vi "Parse Coords.vi"(8 "error in (no error)":errorcluster, 10 "Read Coordinates":path, 11 "Stage Actor.lvlib:Stage.lvclass":refnum<class "Stage.lvclass">) -> (0 "error out":errorcluster, 3 "Stage Actor.lvlib:Stage.lvclass":refnum<class "Stage.lvclass">)   [LabVIEW 2018, in "Stage Actor.lvlib" / "Stage.lvclass"]
uses:
  Stage.lvclass
  Stage.lvclass/Stage.ctl
  <vilib>/Utility/file.llb/Read Delimited Spreadsheet (string).vi
  Stage Actor.lvlib
  <instrlib>/Zaber A Series/Zaber A Series.lvlib
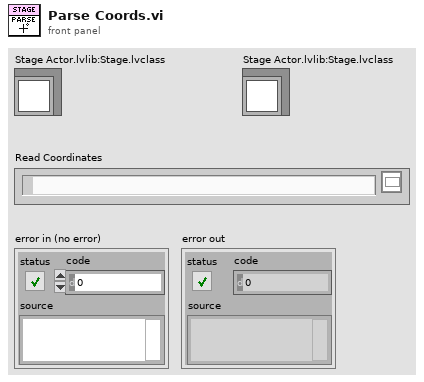
[diagram p1: front panel]
types:
  T1 = enum32{"invalid app kind", "Development System", "Run Time System", "Student Edition", "Embedded LabVIEW", "Evaluation", "Custom"}
  T2 = cluster{"XY":dbl[][], "Theta Phi":dbl[][], "Current Tool":i16[], "Speed":dbl[], "Feeder State":bool[], "Z":dbl[]}
  T3 = cluster{"Current Tool":i16, "Speed":dbl, "Feeder State":bool, "Z":dbl, "XY":dbl[], "Theta Phi":dbl[]}
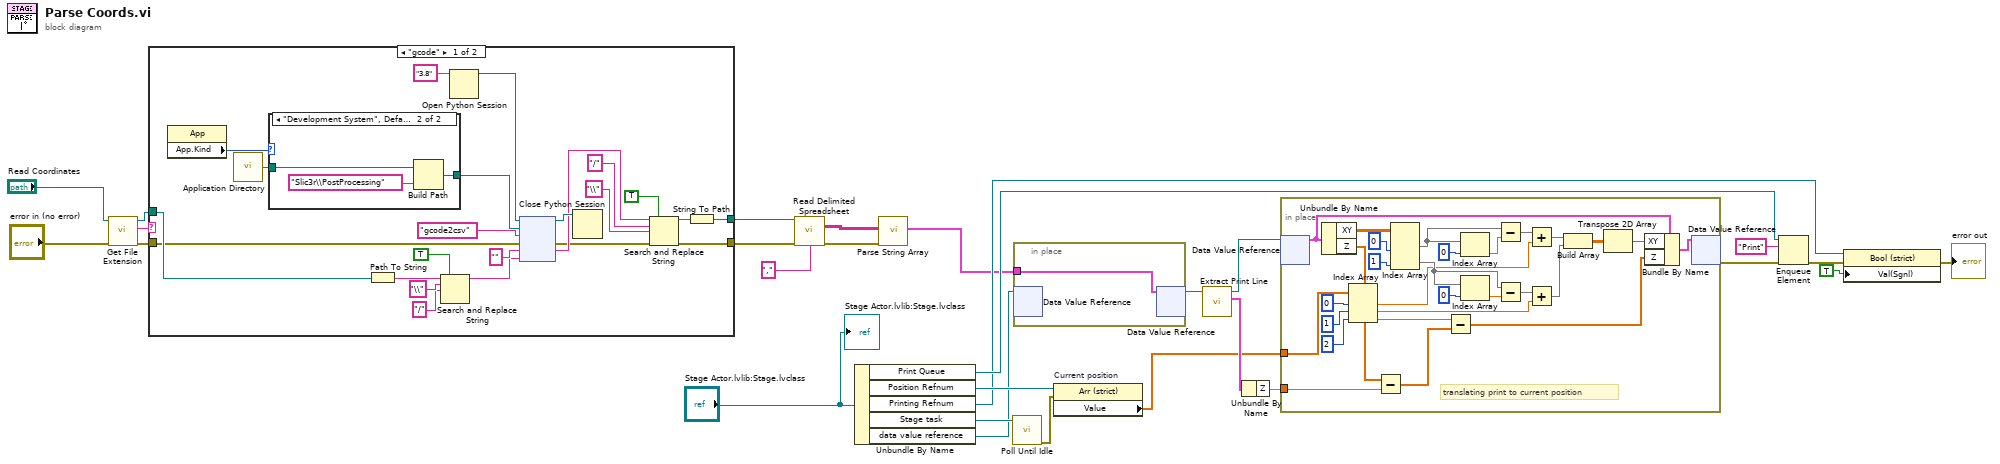
[diagram p0: block diagram]
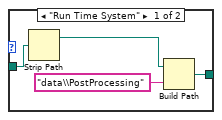
[diagram p2: hidden frame]
diagram:
  n1 = call <vilib>:"Get File Extension.vi"("error in (no error)"="error in (no error)", "file"="Read Coordinates") -> ("error out"=w19:errorcluster, "lowercase file extension"=w21:string, "dup file"=w20:path)  [unwired: 5 in, 2 out]
  n2 = case shown="\"gcode\"" w21 {
    tunnel: w20 -> [w48 w60]
    tunnel: [w35 w60] -> w28
    tunnel: [w33 w59] -> w24
    tunnel: w19 -> [w32 w59]
    frame "gcode" {
      n3 = property class="App"() -> ("App.Kind"=w31:T1)  [unwired: 2 in, 2 out]
      n4 = call <vilib>:"Application Directory.vi"() -> ("Application Directory"=w30:path)
      n5 = case shown="\"Development System\", Default" w31 {
        tunnel: w30 -> [w55 w57]
        tunnel: [w52 w56] -> w29
        frame "Run Time System" {
          n6 = Strip Path(path=w55) -> (stripped path=w53:path)  [unwired: 1 out]
          n7 = Build Path(base path=w53, name or relative path="data\\PostProcessing") -> (appended path=w52:path)
        }
        frame "Development System", Default {
          n8 = Build Path(base path=w57, name or relative path="Slic3r\\PostProcessing") -> (appended path=w56:path)
        }
      }
      n9 = Path To String(path=w48) -> (string=w45:string)
      n10 = Search and Replace String(replace all?=TRUE ("replace all? (F)"), input string=w45, search string="\\", replace string="/" ("replace string (\"\")")) -> (result string=w42:string)  [unwired: 4 in, 3 out]
      n11 = Open Python Session(python version="3.8" ("Python version")) -> (session out=w51:refnum<k35>)  [unwired: 2 in, 1 out]
      n12 = node(w51, w29, "gcode2csv" ("function name"), w32, "", w42) -> (w49:refnum<k35>, w34:errorcluster, w40:string)  [unwired: 1 in, 2 out]
      n13 = Close Python Session(session in=w49) -> ()  [unwired: 1 in, 1 out]
      n14 = Search and Replace String(replace all?=TRUE ("replace all? (F)"), input string=w40, search string="/", replace string="\\" ("replace string (\"\")"), error in=w34) -> (result string=w39:string, error out=w33:errorcluster)  [unwired: 3 in, 2 out]
      n15 = String To Path(string=w39) -> (path=w35:path)
    }
    frame "csv", Default {
    }
  }
  n16 = call-poly <vilib>:"Read Delimited Spreadsheet.vi"("file path (dialog if empty)"=w28, "error in (no error)"=w24, "delimiter (\\t)"="," ("delimiter (\\t)")) -> ("all rows"=w27:string[][], "error out"=w23:errorcluster)  [unwired: 7 in, 4 out]
  n17 = Unbundle By Name("Stage Actor.lvlib:Stage.lvclass") -> ("Print Queue"=w25:refnum<queue>, "Position Refnum"=w16:refnum<vi>, "Printing Refnum"=w14:refnum<vi>, "Stage task"=w11:refnum<visa-resource-name>, "data value reference"=w8:refnum<data-value>)
  n18 = call "Parse String Array.vi"("error in (no error)"=w23, "String XYZ"=w27) -> ("Line Data"=w4:T2)  [unwired: 8 in, 1 out]
  n19 = call <instrlib>:"Poll Until Idle.vi"("VISA resource name"=w11) -> ("error out"=w10:errorcluster)  [unwired: 9 in, 1 out]
  n20 = in-place {
    in-place-border: w4 -> [w61]
    n21 = in-place-dvr #1(w8) -> ()  [unwired: 2 out]
    n22 = in-place-dvr #1(w61) -> (w3:refnum<data-value>)  [unwired: 1 out]
  }
  n23 = property on="Current position" class="Arr (strict)"(reference=w16, error in=w10) -> ("Value"=w5:dbl[])  [unwired: 2 out]
  n24 = call "Extract Print Line.vi"("data value reference"=w3) -> ("Current Line"=w9:T3, "data value reference"=w1:refnum<data-value>)  [unwired: 8 in, 1 out]
  n25 = Unbundle By Name(w9) -> ("Z"=w6:dbl)
  n26 = in-place {
    in-place-border: w6 -> [w72]
    in-place-border: w5 -> [w69]
    # "translating print to current position"
    n27 = in-place-dvr #2(w1) -> (w64:T2)  [unwired: 1 out]
    n28 = Unbundle By Name(w64) -> ("XY"=w89:dbl[][], "Z"=w81:dbl[])
    n29 = Index Array(array=w69, index #1=0 ("index"), index #2=1 ("index"), index #3=2 ("index")) -> (element #1=w76:dbl, element #2=w62:dbl, element #3=w75:dbl)
    n30 = Subtract(x=w81, y=w72) -> (x-y=w82:dbl[])
    n31 = Index Array(array=w89, index (col) #1=0 ("disabled index (col)"), index (col) #2=1 ("index (col)")) -> (element #1=w83:dbl[], element #2=w86:dbl[])  [unwired: 2 in]
    n32 = Subtract(x=w75, y=w82) -> (x-y=w63:dbl[])
    n33 = Index Array(array=w83, index=0) -> (element=w84:dbl)
    n34 = Index Array(array=w86, index=0) -> (element=w85:dbl)
    n35 = Subtract(x=w83, y=w84) -> (x-y=w87:dbl[])
    n36 = Subtract(x=w86, y=w85) -> (x-y=w88:dbl[])
    n37 = Add(x=w87, y=w76) -> (x+y=w77:dbl[])
    n38 = Add(x=w88, y=w62) -> (x+y=w78:dbl[])
    n39 = Build Array(w77, w78) -> (w79:dbl[][])
    n40 = Transpose 2D Array(2D array=w79) -> (transposed array=w80:dbl[][])
    n41 = Bundle By Name(cluster=w64, "XY"=w80, "Z"=w63) -> (w65:T2)
    n42 = in-place-dvr #2(w65) -> (w2:errorcluster)  [unwired: 1 out]
  }
  n43 = Enqueue Element(queue=w25, element="Print" ("Task"), error in (no error)=w2) -> (error out=w13:errorcluster)  [unwired: 1 in, 2 out]
  n44 = property class="Bool (strict)"(reference=w14, error in=w13, "Val(Sgnl)"=TRUE) -> (error out=→"error out":errorcluster)  [unwired: 1 out]
  "Stage Actor.lvlib:Stage.lvclass" <- "Stage Actor.lvlib:Stage.lvclass"
